vi "state_machine_interupt_example - solution.vi"() -> ()   [LabVIEW 2013]
panel:
  out "Stage":string
  in  "Emergency Stop":bool
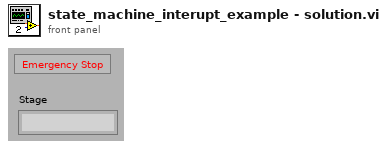
[diagram p1: front panel]
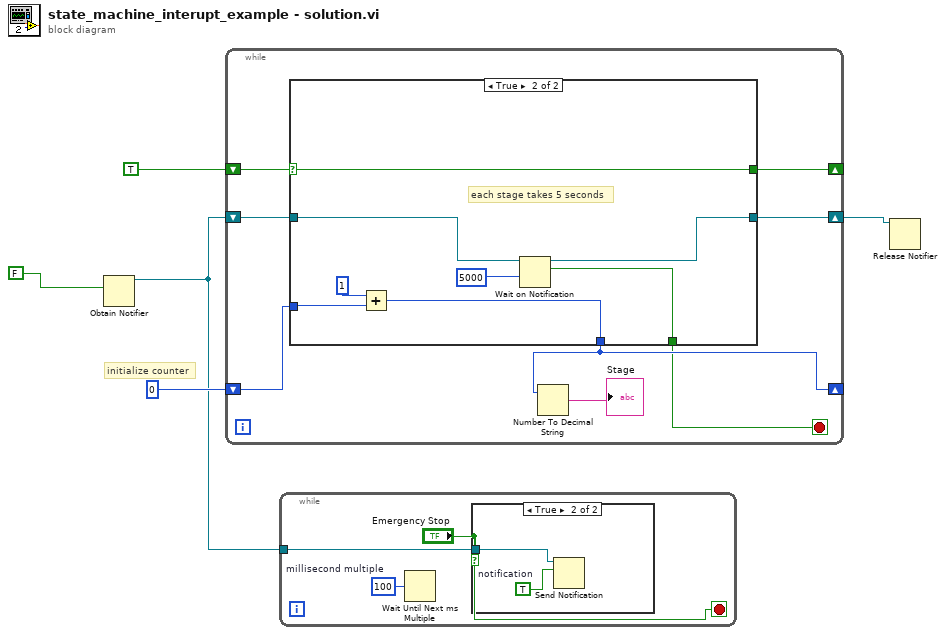
[diagram p0: block diagram]
diagram:
  # "initialize counter"
  n1 = Obtain Notifier(notification data type=FALSE) -> (notifier out=w2:refnum<notifier>)  [unwired: 3 in, 2 out]
  n2 = while {
    shift-right: [w12] -> _
    shift-left: TRUE -> [w13]
    shift-right: [w9] -> _
    shift-left: 0 -> [w11]
    shift-right: [w7] -> w1
    shift-left: w2 -> [w8]
    stop <- w6 stop-if-true
    n3 = case shown="True" w13 {
      selector: w13 -> [w16 w24]
      tunnel: [w16 w24] -> w12
      tunnel: w11 -> [w15 w23]
      tunnel: [w15 w22] -> w9
      tunnel: w8 -> [w14 w20]
      tunnel: [w14 w18] -> w7
      tunnel: [_ w17] -> w6
      frame False {
      }
      frame True {
        # "each stage takes 5 seconds"
        n4 = Add(x=1, y=w23) -> (x+y=w22:i32)
        n5 = Wait on Notification(notifier=w20, timeout in ms (-1)=u32 5000 ("milliseconds to wait")) -> (notifier out=w18:refnum<notifier>, notification=w17:bool)  [unwired: 2 in, 2 out]
      }
    }
    n6 = Number To Decimal String(number=w9) -> (decimal integer string=→"Stage":string)  [unwired: 1 in]
  }
  n7 = while {
    tunnel: w2 -> [w27]
    stop <- "Emergency Stop" stop-if-true
    w26 = u32 100  # millisecond multiple
    n8 = Wait Until Next ms Multiple(millisecond multiple=w26) -> ()  [unwired: 1 out]
    n9 = case shown="True" "Emergency Stop" {
      tunnel: w27 -> [_ w29]
      frame False {
      }
      frame True {
        w28 = TRUE  # notification
        n10 = Send Notification(notification=w28, notifier=w29) -> ()  [unwired: 1 in, 2 out]
      }
    }
  }
  n11 = Release Notifier(notifier=w1) -> ()  [unwired: 2 in, 3 out]
